vi "_wmg_ReportConfigDivided@.vi"(1 "Input":string="TDD11\t1\t1\t0@TDD22\t2\t1\t0@SDD21\t3\t1\t0@SDD22\t4\t1\t0@SCD21\t5\t1\t0@SCD22\t6\t1\t0@SCC11\t7\t1\t0@NEXT\t8\t1\t0@FEXT\t9\t1\t0@") -> (0 "Output":string[][](array[string]))   [LabVIEW 2011]
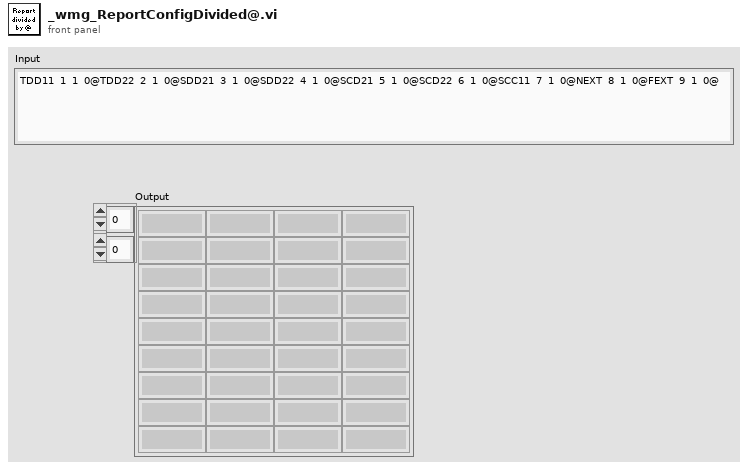
[diagram p1: front panel]
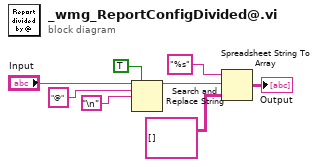
[diagram p0: block diagram]
diagram:
  n1 = Search and Replace String(replace all?=TRUE ("替换全部？(F)"), input string="Input", search string="@" ("搜索字符串"), replace string="\n") -> (result string=w4:string)  [unwired: 4 in, 3 out]
  n2 = Spreadsheet String To Array(format string="%s" ("格式字符串"), spreadsheet string=w4, array type (2D Dbl)=string[][] []) -> (array=→"Output":string[][])  [unwired: 1 in]
